vi "Rinocloud_HTTP_append.vi"(5 "error in (no error)":errorcluster, 7 "chunk":string, 8 "ID":string) -> (0 "error out":errorcluster, 2 "body":string, 3 "headers":string)   [LabVIEW 2013]
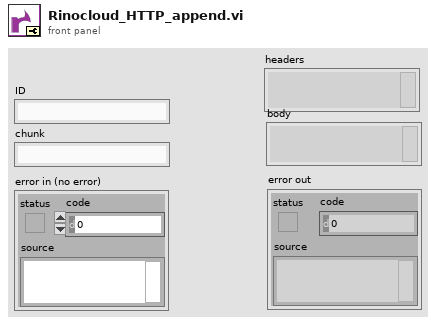
[diagram p1: front panel]
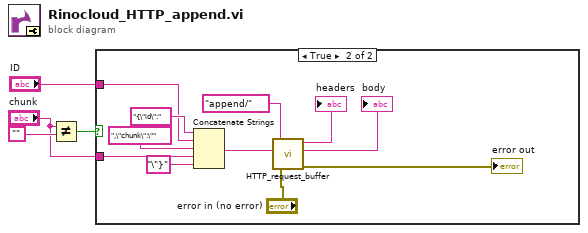
[diagram p0: block diagram]
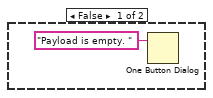
[diagram p2: hidden frame]
diagram:
  n1 = Not Equal?(x="chunk", y="") -> (x != y?=w3:bool)
  n2 = case shown="True" w3 {
    tunnel: "ID" -> [_ w13]
    tunnel: "chunk" -> [_ w12]
    frame False {
      n3 = One Button Dialog(message="Payload is empty. ") -> ()  [unwired: 1 in, 1 out]
    }
    frame True {
      n4 = Concatenate Strings("{\"id\":" ("string"), w13, ",\"chunk\":\"" ("string"), w12, "\"}" ("string")) -> (w10:string)
      n5 = call "HTTP_request_buffer.vi"("error in (no error)"="error in (no error)", "JSON payload"=w10, "Endpoint"="append/") -> ("error out"=→"error out":errorcluster, "body"=→"body":string, "headers"=→"headers":string)  [unwired: 2 in]
    }
  }
